vi "Rotate Angle in Degrees (Array).vi"(7 "output range (-180 to 180)":T1=enum."-180 to 180", 9 "ccw rotation (deg)":dbl, 11 "angles in (deg)":dbl[](array[numeric])) -> (3 "angles out (deg)":dbl[](array[numeric]))   [LabVIEW 2017, in "NI_Robotics Utilities.lvlib"]
doc: "This VI is deprecated. Use <vi.lib>\\Analysis\\coordinate.llb\\Angle Rotation.vi instead."
uses:
  <vilib>/robotics/Utilities/NI_Robotics Utilities.lvlib
  <vilib>/robotics/Utilities/Angle Range_Degrees.ctl
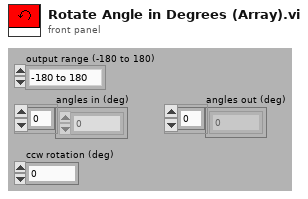
[diagram p1: front panel]
types:
  T1 = typedef "NI_Robotics Utilities.lvlib/Angle Range_Degrees.ctl" = enum16{"none", "-180 to 180", "0 to 360"}
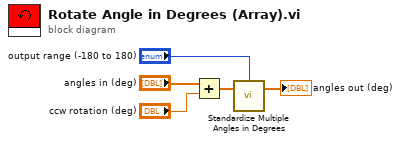
[diagram p0: block diagram]
diagram:
  n1 = Add(x="angles in (deg)", y="ccw rotation (deg)") -> (x+y=w3:dbl[])
  n2 = call <vilib>:"Standardize Multiple Angles in Degrees.vi"("angles in (deg)"=w3, "range (-180 to 180)"="output range (-180 to 180)") -> ("angles out (deg)"=→"angles out (deg)":dbl[])  [unwired: 3 in]
